vi "Ocean-Multi-shot-test.vi"() -> ()   [LabVIEW 2022 SP3]
panel:
  in  "Numeric":i32
  in  "Integration Time (us)":dbl=10000.0
  out "Number of Spectrometers":i32
  out "?":T1(graph)
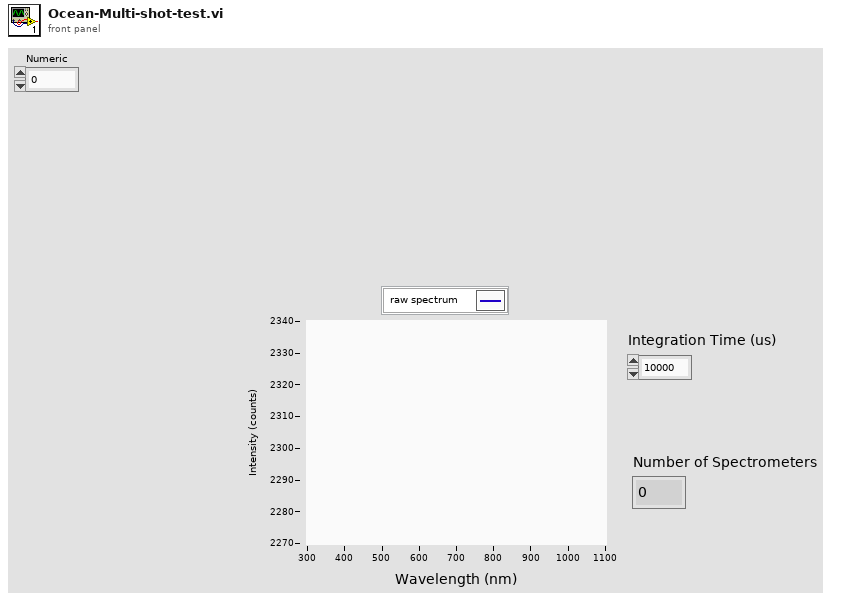
[diagram p1: front panel]
types:
  T1 = cluster{"WL Values":dbl[], "Spectrum Values":dbl[]}
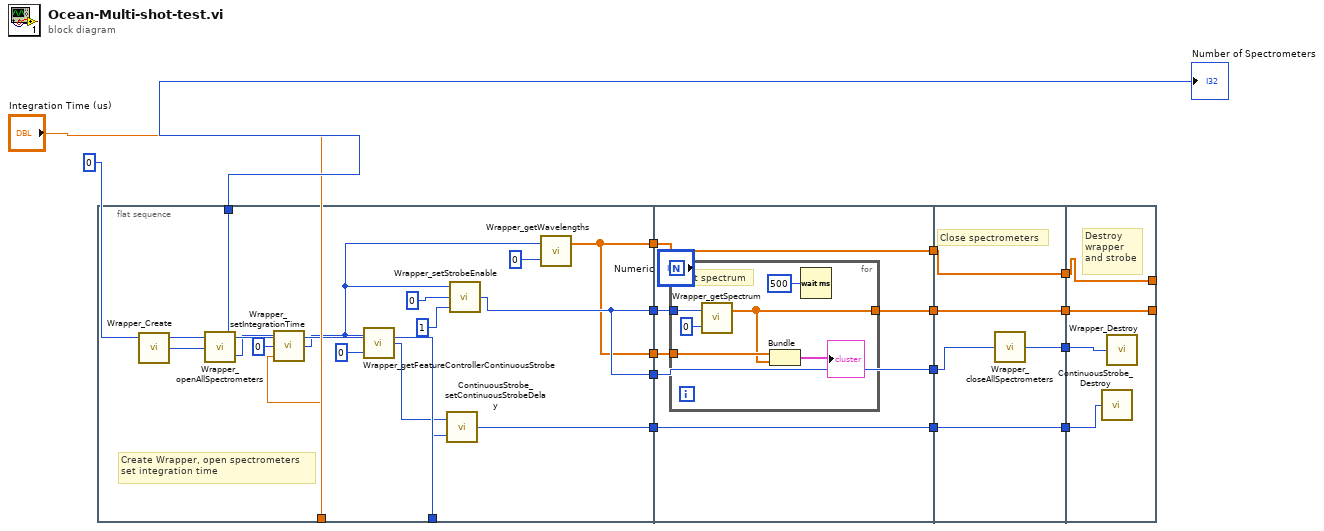
[diagram p0: block diagram]
diagram:
  n1 = flat-sequence {
    tunnel: [w22] -> w16
    tunnel: [w21] -> w15
    tunnel: [w21] -> w14
    tunnel: [w17] -> w13
    tunnel: "Integration Time (us)" -> [w20]
    tunnel: [w19] -> w3
    tunnel: 0 ("Continuous \nStrobe Delay") -> [w18]
    tunnel: [w17] -> w12
    tunnel: [w38] -> w11
    tunnel: w16 -> [w38]
    tunnel: w15 -> [w37]
    tunnel: w14 -> [w36]
    tunnel: [w36] -> w10
    tunnel: w13 -> [w35]
    tunnel: [w35] -> w9
    tunnel: [w34] -> w8
    tunnel: w12 -> [w32]
    tunnel: [w49] -> w7
    tunnel: w11 -> [w49]
    tunnel: w10 -> [w48]
    tunnel: [w47] -> w6
    tunnel: [w46] -> w5
    tunnel: w9 -> [w46]
    tunnel: [w45] -> w4
    tunnel: w8 -> [w45]
    tunnel: w7 -> [w53]
    tunnel: w6 -> [w52]
    tunnel: [w51] -> _
    tunnel: w5 -> [w51]
    tunnel: [w50] -> _
    tunnel: w4 -> [w50]
    frame #0 {
      # "Create Wrapper, open spectrometers\nset integration time"
      n2 = call "Wrapper_Create.vi"() -> ("Wrapper"=w31:u32)
      n3 = call "Wrapper_openAllSpectrometers.vi"("Wrapper In"=w31) -> ("Number of Spectrometers"=w19:i32, "Wrapper Out"=w25:u32)
      n4 = call "Wrapper_setIntegrationTime.vi"("Integration Time"=w20, "Spectrometer Index"=0 ("Index"), "Wrapper In"=w25) -> ("Wrapper Out"=w23:u32)
      n5 = call "Wrapper_getFeatureControllerContinuousStrobe.vi"("Index"=0, "Wrapper"=w23) -> ("ContinuousStrobe"=w28:u32)
      n6 = call "ContinuousStrobe_setContinuousStrobeDelay.vi"("delay"=w18, "ContinuousStrobe In"=w28) -> ("ContinuousStrobe Out"=w22:u32)
      n7 = call "Wrapper_setStrobeEnable.vi"("On/Off"=1, "Index"=0, "Wrapper In"=w23) -> ("Wrapper Out"=w21:u32)
      n8 = call "Wrapper_getWavelengths.vi"("Index"=0, "Wrapper"=w23) -> ("WL Values"=w17:dbl[])  [unwired: 1 out]
    }
    frame #1 {
      n9 = for {
        N: "Numeric" -> [_]
        tunnel: w37 -> [w44]
        tunnel: [w41] -> w34
        tunnel: w32 -> [w42]
        # "Get spectrum"
        n10 = call "Wrapper_getSpectrum.vi"("Index"=0, "Wrapper"=w44) -> ("Spectrum Values"=w41:dbl[])  [unwired: 1 out]
        n11 = Bundle("WL Values"=w42, "Spectrum Values"=w41) -> (→"?":T1)  [unwired: 1 in]
        n12 = Wait (ms)(milliseconds to wait=u32 500) -> ()  [unwired: 1 out]
      }
    }
    frame #2 {
      # "Close spectrometers"
      n13 = call "Wrapper_closeAllSpectrometers.vi"("Wrapper In"=w48) -> ("Wrapper Out"=w47:u32)
    }
    frame #3 {
      # "Destroy \nwrapper \nand strobe"
      n14 = call "ContinuousStrobe_Destroy.vi"("ContinuousStrobe"=w53) -> ()
      n15 = call "Wrapper_Destroy.vi"("Wrapper"=w52) -> ()
    }
  }
  "Number of Spectrometers" <- w3
